vi "Ma move.vi"(1 "Color":i32, 2 "Array Position":cluster{"Row":i32, "Column":i32}, 3 "Chess Array":i32[][](array[numeric])=[[140, 130, 120, 110, 100, 111, 121, 131, 141], [-1, -1, -1, -1, -1, -1, -1, -1, -1], [-1, 150, -1, -1, -1, -1, -1, 151, -1], [160, -1, 161, -1, 162, -1, 163, -1, 164], [-1, -1, -1, -1, -1, -1, -1, -1, -1], [-1, -1, -1, -1, -1, -1, -1, -1, -1], [260, -1, 261, -1, 262, -1, 263, -1, 264], [-1, 250, -1, -1, -1, -1, -1, 251, -1], [-1, -1, -1, -1, -1, -1, -1, -1, -1], [240, 230, 220, 210, 200, 211, 221, 231, 241]]) -> (0 "Ma move":cluster{i32, i32}[](array[cluster]))   [LabVIEW 2009]
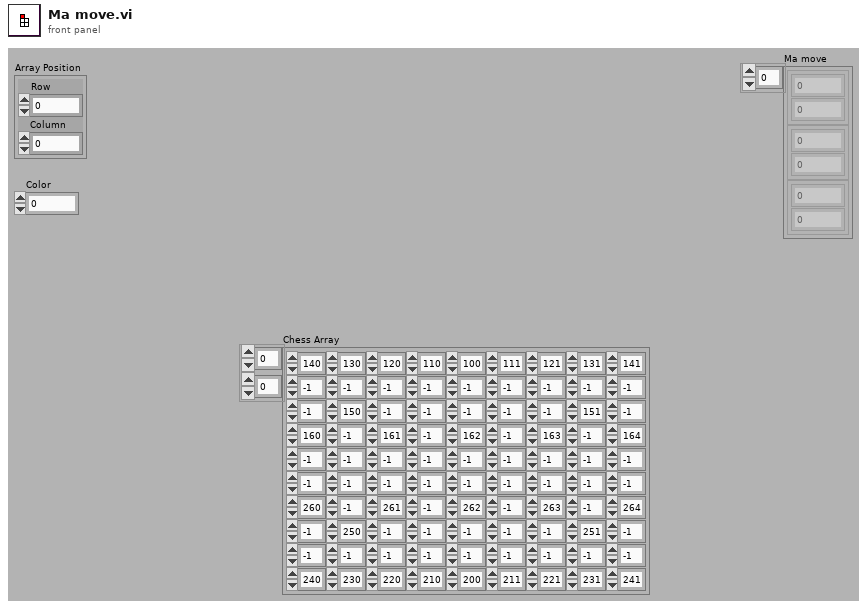
[diagram p1: front panel]
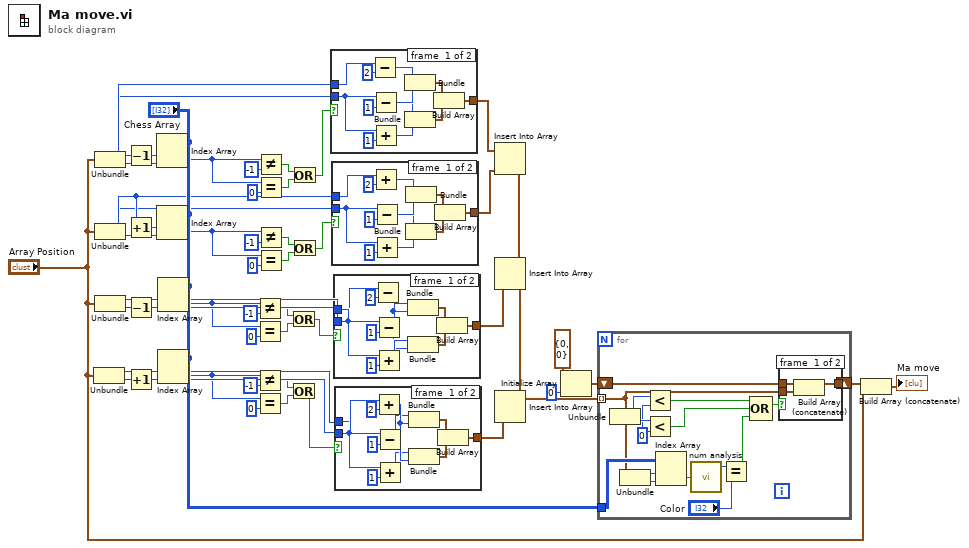
[diagram p0: block diagram]
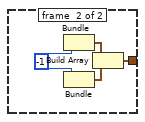
[diagram p3: hidden frame]
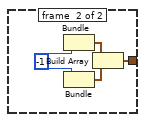
[diagram p4: hidden frame]
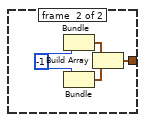
[diagram p5: hidden frame]
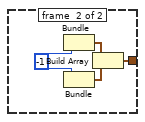
[diagram p6: hidden frame]
diagram:
  n1 = Unbundle("Array Position") -> ("Row"=w38:i32, "Column"=w44:i32)
  n2 = Unbundle("Array Position") -> ("Row"=w50:i32, "Column"=w47:i32)
  n3 = Unbundle("Array Position") -> ("Row"=w46:i32, "Column"=w42:i32)
  n4 = Unbundle("Array Position") -> ("Row"=w40:i32, "Column"=w45:i32)
  n5 = Decrement(x=w50) -> (x-1=w48:i32)
  n6 = Increment(x=w46) -> (x+1=w43:i32)
  n7 = Decrement(x=w45) -> (x-1=w41:i32)
  n8 = Increment(x=w44) -> (x+1=w39:i32)
  n9 = Index Array(array="Chess Array", index (row)=w48, index (col)=w47) -> (element=w36:i32)
  n10 = Index Array(array="Chess Array", index (row)=w43, index (col)=w42) -> (element=w26:i32)
  n11 = Index Array(array="Chess Array", index (row)=w40, index (col)=w41) -> (element=w17:i32)
  n12 = Index Array(array="Chess Array", index (row)=w38, index (col)=w39) -> (element=w16:i32)
  n13 = Not Equal?(x=w17, y=-1) -> (x != y?=w23:bool)
  n14 = Equal?(x=w17, y=0) -> (x = y?=w22:bool)
  n15 = Not Equal?(x=w16, y=-1) -> (x != y?=w20:bool)
  n16 = Equal?(x=w16, y=0) -> (x = y?=w21:bool)
  n17 = Not Equal?(x=w36, y=-1) -> (x != y?=w34:bool)
  n18 = Equal?(x=w36, y=0) -> (x = y?=w33:bool)
  n19 = Not Equal?(x=w26, y=-1) -> (x != y?=w30:bool)
  n20 = Equal?(x=w26, y=0) -> (x = y?=w31:bool)
  n21 = Or(x=w23, y=w22) -> (x .or. y?=w15:bool)
  n22 = Or(x=w20, y=w21) -> (x .or. y?=w14:bool)
  n23 = Or(x=w34, y=w33) -> (x .or. y?=w32:bool)
  n24 = Or(x=w30, y=w31) -> (x .or. y?=w27:bool)
  n25 = case shown="False" w32 {
    tunnel: w50 -> [w61 _]
    tunnel: w47 -> [w56 _]
    tunnel: [w51 w63] -> w13
    frame #0 {
      n26 = Subtract(x=w61, y=2) -> (x-y=w55:i32)
      n27 = Subtract(x=w56, y=1) -> (x-y=w59:i32)
      n28 = Add(x=w56, y=1) -> (x+y=w54:i32)
      n29 = Bundle(w55, w59) -> (w53:cluster{i32, i32})  [unwired: 1 out]
      n30 = Bundle(w55, w54) -> (w52:cluster{i32, i32})  [unwired: 1 out]
      n31 = Build Array(w53, w52) -> (w51:cluster{i32, i32}[])
    }
    frame #1 {
      w62 = -1 ("y")
      n32 = Bundle("y"=w62, "y"=w62) -> (w65:cluster{"y":i32, "y":i32})  [unwired: 1 out]
      n33 = Bundle("y"=w62, "y"=w62) -> (w64:cluster{"y":i32, "y":i32})  [unwired: 1 out]
      n34 = Build Array(w65, w64) -> (w63:cluster{"y":i32, "y":i32}[])
    }
  }
  n35 = case shown="False" w27 {
    tunnel: w46 -> [w76 _]
    tunnel: w42 -> [w71 _]
    tunnel: [w66 w78] -> w12
    frame #0 {
      n36 = Add(x=w76, y=2) -> (x+y=w70:i32)
      n37 = Subtract(x=w71, y=1) -> (x-y=w74:i32)
      n38 = Add(x=w71, y=1) -> (x+y=w69:i32)
      n39 = Bundle(w70, w74) -> (w68:cluster{i32, i32})  [unwired: 1 out]
      n40 = Bundle(w70, w69) -> (w67:cluster{i32, i32})  [unwired: 1 out]
      n41 = Build Array(w68, w67) -> (w66:cluster{i32, i32}[])
    }
    frame #1 {
      w77 = -1 ("y")
      n42 = Bundle("y"=w77, "y"=w77) -> (w80:cluster{"y":i32, "y":i32})  [unwired: 1 out]
      n43 = Bundle("y"=w77, "y"=w77) -> (w79:cluster{"y":i32, "y":i32})  [unwired: 1 out]
      n44 = Build Array(w80, w79) -> (w78:cluster{"y":i32, "y":i32}[])
    }
  }
  n45 = case shown="False" w15 {
    tunnel: w40 -> [w85 _]
    tunnel: w45 -> [w84 _]
    tunnel: [w86 w93] -> w10
    frame #0 {
      n46 = Subtract(x=w84, y=2) -> (x-y=w81:i32)
      n47 = Subtract(x=w85, y=1) -> (x-y=w83:i32)
      n48 = Add(x=w85, y=1) -> (x+y=w82:i32)
      n49 = Bundle(w83, w81) -> (w88:cluster{i32, i32})  [unwired: 1 out]
      n50 = Bundle(w82, w81) -> (w87:cluster{i32, i32})  [unwired: 1 out]
      n51 = Build Array(w88, w87) -> (w86:cluster{i32, i32}[])
    }
    frame #1 {
      w92 = -1 ("y")
      n52 = Bundle("y"=w92, "y"=w92) -> (w95:cluster{"y":i32, "y":i32})  [unwired: 1 out]
      n53 = Bundle("y"=w92, "y"=w92) -> (w94:cluster{"y":i32, "y":i32})  [unwired: 1 out]
      n54 = Build Array(w95, w94) -> (w93:cluster{"y":i32, "y":i32}[])
    }
  }
  n55 = case shown="False" w14 {
    tunnel: w38 -> [w99 _]
    tunnel: w44 -> [w100 _]
    tunnel: [w101 w108] -> w8
    frame #0 {
      n56 = Add(x=w100, y=2) -> (x+y=w98:i32)
      n57 = Subtract(x=w99, y=1) -> (x-y=w97:i32)
      n58 = Add(x=w99, y=1) -> (x+y=w96:i32)
      n59 = Bundle(w97, w98) -> (w103:cluster{i32, i32})  [unwired: 1 out]
      n60 = Bundle(w96, w98) -> (w102:cluster{i32, i32})  [unwired: 1 out]
      n61 = Build Array(w103, w102) -> (w101:cluster{i32, i32}[])
    }
    frame #1 {
      w107 = -1 ("y")
      n62 = Bundle("y"=w107, "y"=w107) -> (w110:cluster{"y":i32, "y":i32})  [unwired: 1 out]
      n63 = Bundle("y"=w107, "y"=w107) -> (w109:cluster{"y":i32, "y":i32})  [unwired: 1 out]
      n64 = Build Array(w110, w109) -> (w108:cluster{"y":i32, "y":i32}[])
    }
  }
  n65 = Insert Into Array(array=w13, new element=w12) -> (w11:cluster{"y":i32, "y":i32}[])  [unwired: 1 in]
  n66 = Insert Into Array(array=w11, new element=w10) -> (w9:cluster{"y":i32, "y":i32}[])  [unwired: 1 in]
  n67 = Insert Into Array(array=w9, new element=w8) -> (w7:cluster{"y":i32, "y":i32}[])  [unwired: 1 in]
  n68 = Initialize Array(cluster{i32, i32} {0, 0} ("Output Cluster"), 0 ("Dimension Size")) -> (w6:cluster{i32, i32}[])
  n69 = for {
    tunnel: w7 -> [w117] mode=indexing
    shift-right: [w119] -> w3
    shift-left: w6 -> [w120]
    tunnel: "Chess Array" -> [w118]
    w124 = 0 ("y")
    n70 = Unbundle(w117) -> ("y"=w126:i32, "y"=w125:i32)
    n71 = Unbundle(w117) -> ("y"=w116:i32, "y"=w115:i32)
    n72 = Less?(x=w126, y=w124) -> (x < y?=w122:bool)
    n73 = Less?(x=w125, y=w124) -> (x < y?=w123:bool)
    n74 = Index Array(array=w118, index (row)=w116, index (col)=w115) -> (element=w114:i32)
    n75 = call "num analysis.vi"("x"=w114) -> ("Color"=w113:i32)  [unwired: 2 out]
    n76 = Equal?(x=w113, y="Color") -> (x = y?=w111:bool)
    n77 = Compound Arithmetic op=OR(w122, w123, w111) -> (w121:bool)
    n78 = case shown="False" w121 {
      tunnel: w120 -> [w129 w130]
      tunnel: [w127 w130] -> w119
      tunnel: w117 -> [w128 _]
      frame #0 {
        n79 = Build Array (concatenate)(w129, w128) -> (w127:cluster{"y":i32, "y":i32}[])
      }
      frame #1 {
      }
    }
  }
  n80 = Build Array (concatenate)(w3, "Array Position") -> (→"Ma move":cluster{"Row":i32, "Column":i32}[])
